vi "_read_yokogawa.vi"(3 "error in":errorcluster, 4 "Bytes to read":u32, 5 "Command to read":string) -> (0 "error out":errorcluster, 2 "Output":string)   [LabVIEW 2013]
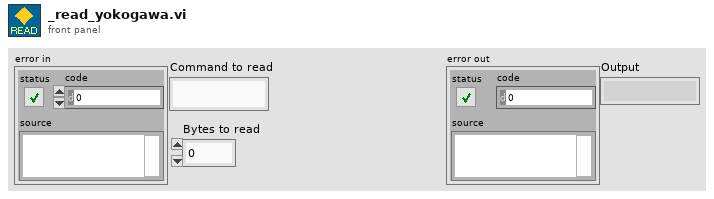
[diagram p1: front panel]
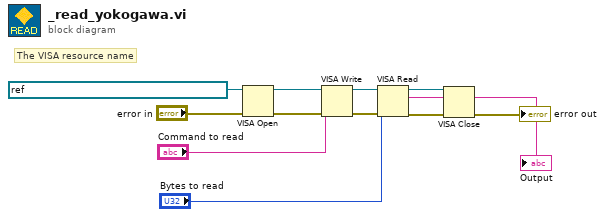
[diagram p0: block diagram]
diagram:
  # "The VISA resource name"
  n1 = VISA Open(error in (no error)="error in", VISA resource name=refnum<visa-resource-name> "USB::0xB21::0x39::91NA15589::INSTR") -> (VISA resource name=w11:refnum<visa-resource-name>, error out=w10:errorcluster)  [unwired: 3 in]
  n2 = VISA Write(VISA resource name=w11, write buffer="Command to read", error in (no error)=w10) -> (VISA resource name out=w5:refnum<visa-resource-name>, error out=w6:errorcluster)  [unwired: 1 out]
  n3 = VISA Read(VISA resource name=w5, byte count="Bytes to read", error in (no error)=w6) -> (VISA resource name out=w4:refnum<visa-resource-name>, read buffer=→"Output":string, error out=w3:errorcluster)  [unwired: 1 out]
  n4 = VISA Close(VISA resource name=w4, error in (no error)=w3) -> (error out=→"error out":errorcluster)
